vi "GetShortcut.vi"(8 "error in (no error)":errorcluster, 11 "text item in":refnum<class "text item.lvclass">) -> (0 "error out":errorcluster, 2 "shortcut":string, 3 "text item out":refnum<class "text item.lvclass">)   [LabVIEW 2009, in "text item.lvclass"]
uses:
  text item.lvclass
  text item.lvclass/text item.ctl
  Text/text.lvclass
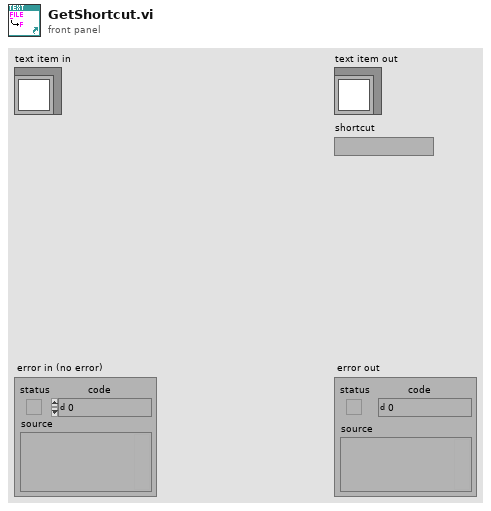
[diagram p1: front panel]
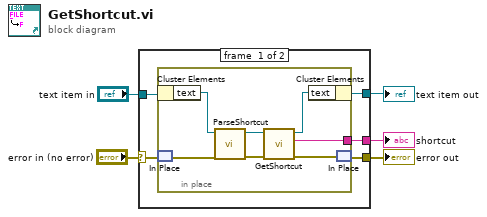
[diagram p0: block diagram]
diagram:
  n1 = case shown="No Error" "error in (no error)" {
    selector: "error in (no error)" -> [w8 w18]
    tunnel: "text item in" -> [w10 w19]
    tunnel: [w9 _] -> w4
    tunnel: [w7 w18] -> w2
    tunnel: [w6 w19] -> w1
    frame #0 {
      n2 = in-place {
        in-place-border: [w15] -> w9
        n3 = in-place-cluster #1(w10) -> ("text"=w14:refnum<class "text.lvclass">)
        n4 = in-place-match #2(w8) -> (w11:errorcluster)
        n5 = call "ParseShortcut.vi"("error in (no error)"=w11, "text in"=w14) -> ("error out"=w16:errorcluster, "text out"=w17:refnum<class "text.lvclass">)  [unwired: 8 in]
        n6 = call "GetShortcut.vi"("error in (no error)"=w16, "text in"=w17) -> ("error out"=w12:errorcluster, "shortcut"=w15:string, "text out"=w13:refnum<class "text.lvclass">)  [unwired: 7 in]
        n7 = in-place-cluster #1("text"=w13) -> (w6:refnum<class "text item.lvclass">)
        n8 = in-place-match #2(w12) -> (w7:errorcluster)
      }
    }
    frame #1 {
    }
  }
  "text item out" <- w1
  "error out" <- w2
  "shortcut" <- w4
